vi "SMTP Email Wrap Subject Field.vi"(1 "Subject in":string) -> (0 "Subject out":string)   [LabVIEW 2012, in "NewNI_SMTPEmail.lvlib"]
doc: "Wraps the encoded Subject field so that it does not exceed the maximum line length as specified in RFC1522."
uses:
  NewNI_SMTPEmail.lvlib
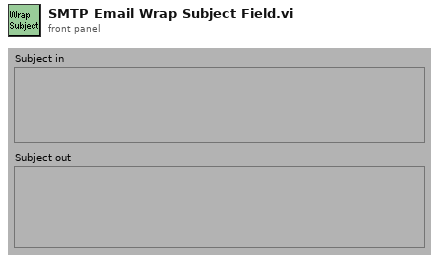
[diagram p1: front panel]
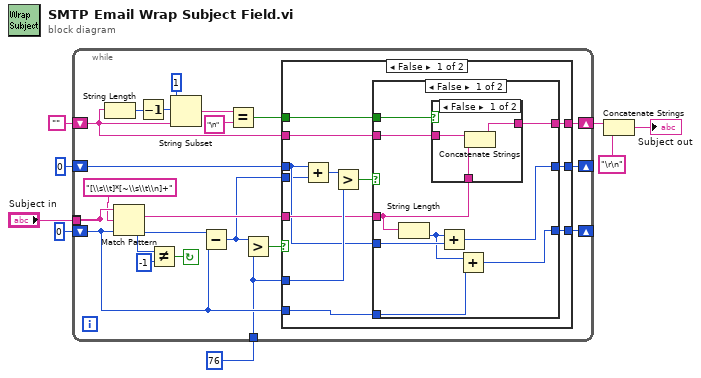
[diagram p0: block diagram]
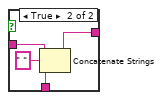
[diagram p2: hidden frame]
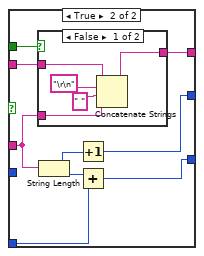
[diagram p3: hidden frame]
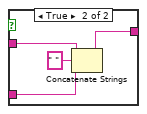
[diagram p4: hidden frame]
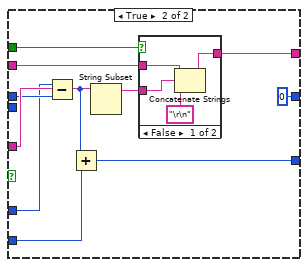
[diagram p5: hidden frame]
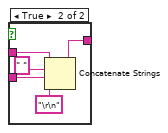
[diagram p6: hidden frame]
diagram:
  n1 = while {
    tunnel: 76 ("y") -> [w10]
    shift-left: "" -> [w11]
    shift-right: [w24] -> w7
    shift-left: 0 -> [w22]
    shift-right: [w21] -> _
    shift-left: 0 -> [w18]
    shift-right: [w20] -> _
    tunnel: "Subject in" -> [w29]
    tunnel: [w29] -> _
    stop <- w27 continue-if-true
    n2 = String Length(string=w11) -> (length=w16:i32)
    n3 = Match Pattern(string=w29, regular expression="[\\s\\t]*[~\\s\\t\\n]+", offset (0)=w18) -> (match substring=w23:string, offset past match=w19:i32)  [unwired: 2 out]
    n4 = Decrement(x=w16) -> (x-1=w15:i32)
    n5 = Not Equal?(x=w19, y=-1) -> (x != y?=w27:bool)
    n6 = String Subset(string=w11, offset (0)=w15, length (rest)=1 ("length")) -> (substring=w14:string)
    n7 = Subtract(x=w19, y=w18) -> (x-y=w12:i32)
    n8 = Equal?(x=w14, y="\n") -> (x = y?=w13:bool)
    n9 = Greater?(x=w12, y=w10) -> (0:w25:bool)
    n10 = case shown="False" w25 {
      tunnel: [w37 w78] -> w24
      tunnel: w23 -> [w38 w85]
      tunnel: w22 -> [w32 w84]
      tunnel: [w34 0] -> w21
      tunnel: [w35 w80] -> w20
      tunnel: w18 -> [w36 w82]
      tunnel: w13 -> [w33 w77]
      tunnel: w12 -> [w31 _]
      tunnel: w11 -> [w30 w76]
      tunnel: w10 -> [w40 w75]
      frame False {
        n11 = Add(x=w32, y=w31) -> (x+y=w41:i32)
        n12 = Greater?(x=w41, y=w40) -> (0:w39:bool)
        n13 = case shown="False" w39 {
          tunnel: w38 -> [w49 w64]
          tunnel: [w50 w65] -> w37
          tunnel: w36 -> [w43 w62]
          tunnel: [w46 w61] -> w35
          tunnel: [w47 w60] -> w34
          tunnel: w33 -> [w45 w59]
          tunnel: w32 -> [w48 _]
          tunnel: w30 -> [w42 w58]
          frame False {
            n14 = String Length(string=w49) -> (length=w44:i32)
            n15 = case shown="False" w45 {
              tunnel: w49 -> [w53 w55]
              tunnel: [w52 w57] -> w50
              tunnel: w42 -> [w51 w54]
              frame False {
                n16 = Concatenate Strings(w51, w53) -> (w52:string)
              }
              frame True {
                n17 = Concatenate Strings(w54, " ", w55) -> (w57:string)
              }
            }
            n18 = Add(x=w44, y=w48) -> (x+y=w47:i32)
            n19 = Add(x=w44, y=w43) -> (x+y=w46:i32)
          }
          frame True {
            n20 = case shown="False" w59 {
              tunnel: w64 -> [w67 w73]
              tunnel: [w68 w72] -> w65
              tunnel: w58 -> [w66 w71]
              frame False {
                n21 = Concatenate Strings(w66, "\r\n", " " ("CRLF"), w67) -> (w68:string)
              }
              frame True {
                n22 = Concatenate Strings(w71, " ", w73) -> (w72:string)
              }
            }
            n23 = String Length(string=w64) -> (length=w63:i32)
            n24 = Increment(x=w63) -> (x+1=w60:i32)
            n25 = Add(x=w63, y=w62) -> (x+y=w61:i32)
          }
        }
      }
      frame True {
        n26 = Subtract(x=w75, y=w84) -> (x-y=w81:i32)
        n27 = Add(x=w81, y=w82) -> (x+y=w80:i32)
        n28 = String Subset(string=w85, length (rest)=w81) -> (substring=w79:string)  [unwired: 1 out]
        n29 = case shown="False" w77 {
          tunnel: w79 -> [w89 w93]
          tunnel: [w88 w92] -> w78
          tunnel: w76 -> [w87 w91]
          frame False {
            n30 = Concatenate Strings(w87, w89, "\r\n") -> (w88:string)
          }
          frame True {
            n31 = Concatenate Strings(w91, " ", w93, "\r\n") -> (w92:string)
          }
        }
      }
    }
  }
  n32 = Concatenate Strings(w7, "\r\n") -> (→"Subject out":string)
